vi "SpotToOvalCoordinates.vi"(4 "Spot":i32[](array[numeric]), 6 "plane":u32) -> (1 "Pos array":i32[][](array[numeric]), 2 "starting y-point":i32, 3 "oval coordinates":i32[](array[numeric]))   [LabVIEW 2009]
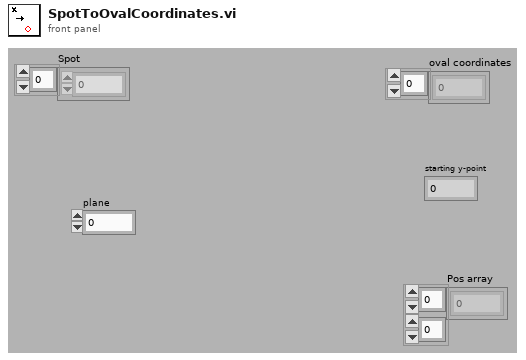
[diagram p1: front panel]
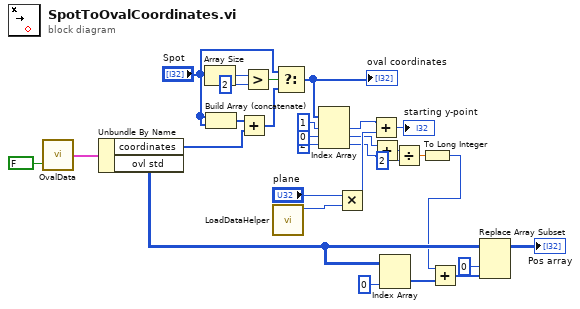
[diagram p0: block diagram]
diagram:
  n1 = call "OvalData.vi"("changed?"=FALSE) -> ("data"=w29:cluster{"coordinates":i32[], "ovl std":i32[][]})  [unwired: 1 in]
  n2 = Unbundle By Name(w29) -> ("coordinates"=w24:i32[], "ovl std"=w12:i32[][])
  n3 = Array Size(array="Spot") -> (size(s)=w28:i32)
  n4 = Build Array (concatenate)("Spot", "Spot") -> (w25:i32[])
  n5 = Add(x=w25, y=w24) -> (x+y=w23:i32[])
  n6 = Greater?(x=w28, y=2) -> (0:w26:bool)
  n7 = call "LoadDataHelper.vi"() -> ("lines"=w19:u32)  [unwired: 7 in, 4 out]
  n8 = Select(t="Spot", s=w26, f=w23) -> (s? t:f=w22:i32[])
  "oval coordinates" <- w22
  n9 = Index Array(array=w22, index #1=1 ("index"), index #2=0 ("index"), index #3=2 ("index")) -> (element #1=w17:i32, element #2=w6:i32, element #3=w5:i32)
  n10 = Multiply(x="plane", y=w19) -> (x*y=w16:u32)
  n11 = Add(x=w17, y=w16) -> (x+y=→"starting y-point":u32)
  n12 = Add(x=w6, y=w5) -> (x+y=w4:i32)
  n13 = Index Array(array=w12, index (col)=0 ("disabled index (col)")) -> (element=w14:i32[])  [unwired: 1 in]
  n14 = Divide(x=w4, y=2) -> (x/y=w2:dbl)
  n15 = To Long Integer(number=w2) -> (32bit integer=w1:i32)
  n16 = Add(x=w1, y=w14) -> (x+y=w13:i32[])
  n17 = Replace Array Subset(array=w12, new element=w13, index (col)=0 ("disabled index (col)")) -> (→"Pos array":i32[][])  [unwired: 1 in]
